vi "Save MATLAB File example.vi"() -> ()   [LabVIEW 2020]
panel:
  in  "delimiter (Tab)":string
  in  "format string":string
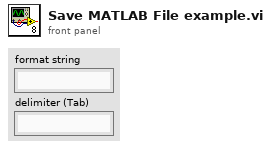
[diagram p1: front panel]
types:
  T1 = enum16{"open", "replace", "create", "open or create", "replace or create", "replace or create with confirmation"}
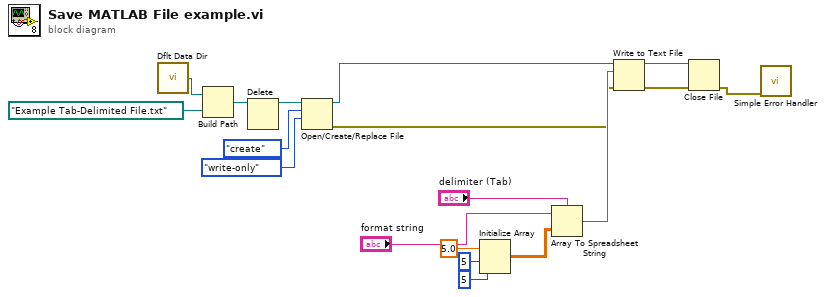
[diagram p0: block diagram]
diagram:
  n1 = call <vilib>:"Dflt Data Dir.vi"() -> ("App:Default Data Directory"=w5:path)
  n2 = Build Path(base path=w5, name or relative path=path "Example Tab-Delimited File.txt" ("default name")) -> (appended path=w7:path)
  n3 = Delete(path (use dialog)=w7) -> (deleted path=w4:path)  [unwired: 4 in, 2 out]
  n4 = Open/Create/Replace File(file path (use dialog)=w4, operation (0:open)=T1."create", access (0:read/write)=enum16{"read/write", "read-only", "write-only"}."write-only") -> (refnum out=w3:refnum<file>, error out=w2:errorcluster)  [unwired: 1 in, 3 out]
  n5 = Initialize Array(5.0 ("element"), 5 ("dimension size"), 5 ("dimension size")) -> (w13:dbl[][])
  n6 = Array To Spreadsheet String(delimiter (Tab)="delimiter (Tab)", array=w13, 3:"format string") -> (spreadsheet string=w12:string)
  n7 = Write to Text File(file (use dialog)=w3, text=w12, error in=w2) -> (refnum out=w18:refnum<file>, error out=w17:errorcluster)  [unwired: 1 in, 1 out]
  n8 = Close File(refnum=w18, error in=w17) -> (error out=w1:errorcluster)  [unwired: 1 out]
  n9 = call <vilib>:"Simple Error Handler.vi"("error in (no error)"=w1) -> ()  [unwired: 1 in, 8 out]
